vi "Read Measurement Name.vi"(8 "error in (no error)":errorcluster, 11 "Measurement in":refnum<class "Measurement.lvclass">) -> (0 "error out":errorcluster, 2 "Measurement Name":string, 3 "Measurement out":refnum<class "Measurement.lvclass">)   [LabVIEW 2026, in "Measurement Actor.lvlib" / "Measurement.lvclass"]
uses:
  Measurement.lvclass
  Measurement.lvclass/Measurement.ctl
  recovery/packages/oglib_file-4.0.1.22-8A89CE420A/File Group 0/user.lib/_OpenG.lib/file/file.llb/Strip Path Extension - String__ogtk.vi
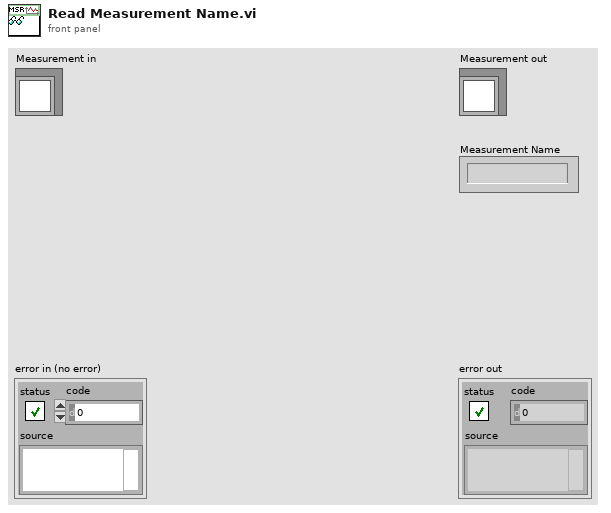
[diagram p1: front panel]
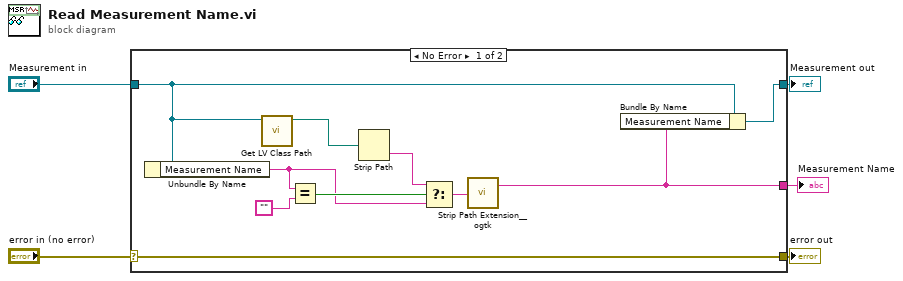
[diagram p0: block diagram]
diagram:
  n1 = case shown="No Error" "error in (no error)" {
    selector: "error in (no error)" -> [w15 w16]
    tunnel: [w15 w16] -> w4
    tunnel: [w6 w17] -> w2
    tunnel: "Measurement in" -> [w7 w17]
    tunnel: [w8 _] -> w1
    frame No Error {
      n2 = Unbundle By Name(w7) -> ("Measurement Name"=w12:string)
      n3 = call <vilib>:"Get LV Class Path.vi"("object"=w7) -> ("class path"=w10:path)  [unwired: 9 in, 1 out]
      n4 = Equal?(x=w12, y="") -> (x = y?=w13:bool)
      n5 = Strip Path(path=w10) -> (name=w11:string)  [unwired: 1 out]
      n6 = Select(t=w11, s=w13, f=w12) -> (s? t:f=w9:string)
      n7 = call-poly "Strip Path Extension__ogtk.vi"("path"=w9) -> ("root"=w8:string)  [unwired: 1 out]
      n8 = Bundle By Name(cluster=w7, "Measurement Name"=w8) -> (w6:refnum<class "Measurement.lvclass">)
    }
    frame Error {
    }
  }
  "error out" <- w4
  "Measurement out" <- w2
  "Measurement Name" <- w1
